vi "EnvMillik.vi"() -> ()   [LabVIEW 2016]
uses:
  <vilib>/addons/database/NI_Database_API.lvlib
panel:
  out "read buffer":string
  in  "stop":bool
  out "error out":errorcluster
  in  "error in (no error)":errorcluster
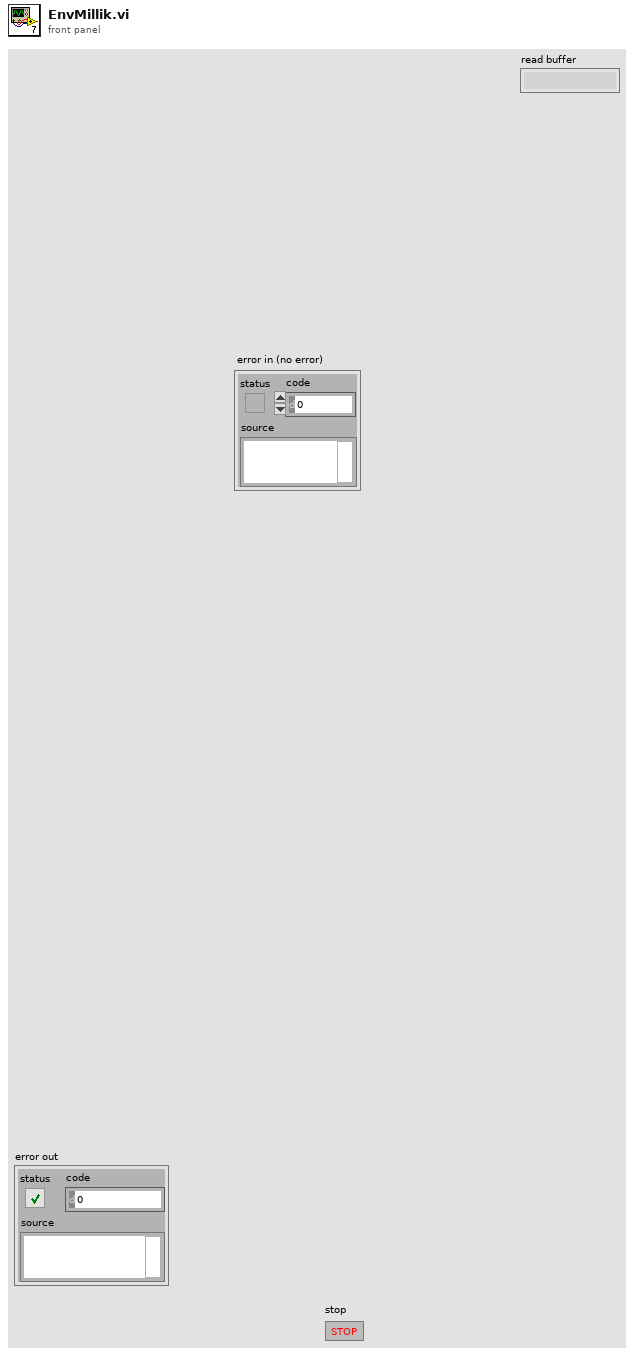
[diagram p1: front panel]
types:
  T1 = typedef "NI_Database_API.lvlib/Conn ObjectReference.ctl" = refnum<k1>
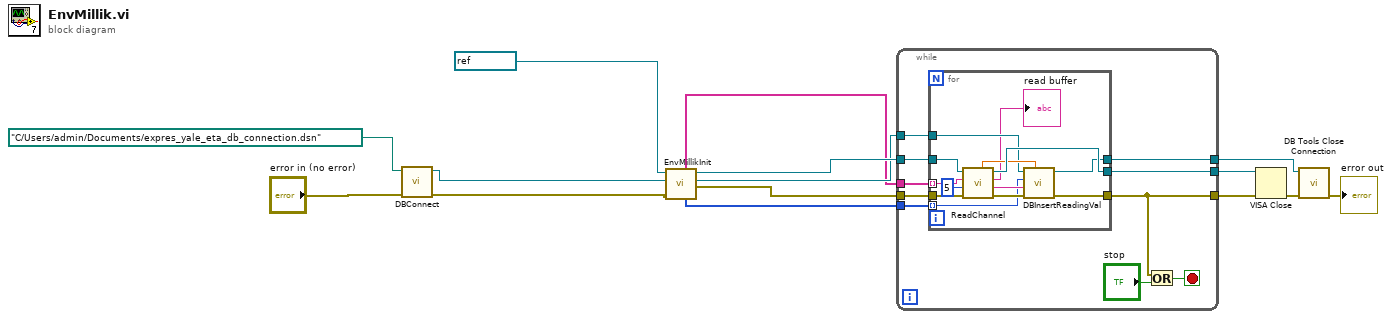
[diagram p0: block diagram]
diagram:
  n1 = call "DBConnect.vi"("error in (no error)"="error in (no error)", "connection path"=path "C:/Users/admin/Documents/expres_yale_eta_db_connection.dsn") -> ("error out"=w13:errorcluster, "db connection out"=w1:T1)  [unwired: 8 in]
  n2 = call "EnvMillikInit.vi"("error in (no error)"=w13, "db connection in"=w1, "VISA Refnum in"=refnum<visa-resource-name> "COM3" ("VISA resource name")) -> ("error out"=w8:errorcluster, "db connection out"=w6:T1, "VISA Refnum out"=w7:refnum<visa-resource-name>, "sensor id array out"=w2:i32[], "channel array out"=w5:string[])  [unwired: 4 in]
  n3 = while {
    tunnel: w5 -> [w22]
    tunnel: w7 -> [w23]
    tunnel: [w25] -> w12
    tunnel: w8 -> [w24]
    tunnel: w6 -> [w19]
    tunnel: [w17] -> w4
    tunnel: [w18] -> w3
    tunnel: w2 -> [w16]
    stop <- w21 stop-if-true
    n4 = for {
      tunnel: w22 -> [w28] mode=indexing
      tunnel: w23 -> [w36]
      tunnel: [w38] -> w25
      tunnel: w24 -> [w37]
      tunnel: w19 -> [w34]
      tunnel: [w32] -> w17
      tunnel: [w31] -> w18
      tunnel: w16 -> [w26] mode=indexing
      n5 = call "ReadChannel.vi"("error in (no error)"=w37, "timeout"=5, "channel"=w28, "VISA Refnum in"=w36) -> ("error out"=w33:errorcluster, "timestamp"=w30:string, "read buffer"=→"read buffer":string, "VISA Refnum out"=w38:refnum<visa-resource-name>, "value"=w35:dbl)  [unwired: 3 in]
      n6 = call "DBInsertReadingVal.vi"("db connection in"=w34, "sensor id"=w26, "timestamp"=w30, "error in (no error)"=w33, "reading value"=w35) -> ("db connection out"=w31:T1, "error out"=w32:errorcluster)  [unwired: 4 in]
    }
    n7 = Or(x=w17, y="stop") -> (x .or. y?=w21:bool)
  }
  n8 = VISA Close(VISA resource name=w12, error in (no error)=w4) -> (error out=w10:errorcluster)
  n9 = call <vilib>:"DB Tools Close Connection.vi"("error in (no error)"=w10, "connection reference"=w3) -> ("error out"=→"error out":errorcluster)  [unwired: 5 in]
